vi "Transaction.vi"(8 "Error In":errorcluster, 9 "Bytes to read (1024)":u32=1024, 10 "Command":string, 11 "VISA resource name":refnum<visa-resource-name>) -> (0 "Error Out":errorcluster, 2 "Response":string, 3 "VISA resource name out":refnum<visa-resource-name>)   [LabVIEW 2013, in "HadCon.lvlib"]
doc: "This VI performs low level command /response formatting.\nThis transaction sends a command and waits for the corresponding response of the instrument."
uses:
  <instrlib>/HadCon/HadCon.lvlib
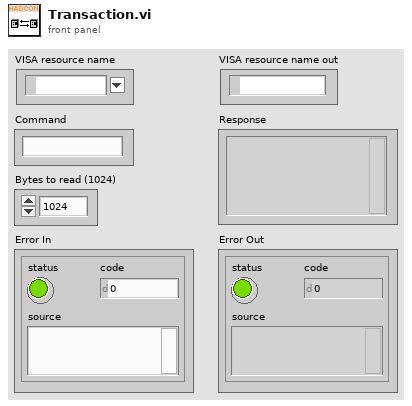
[diagram p1: front panel]
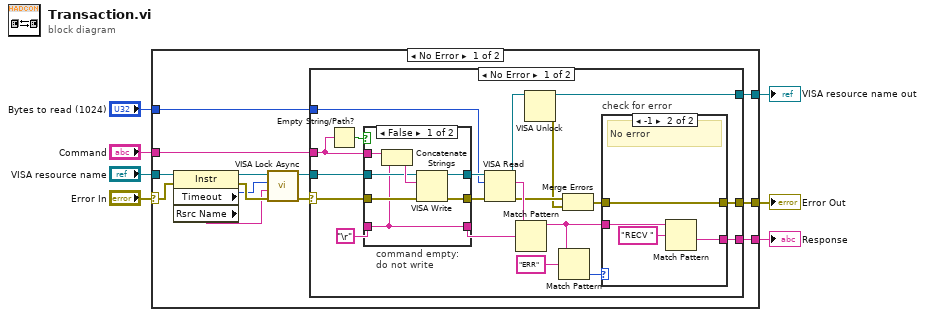
[diagram p0: block diagram]
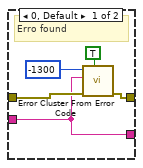
[diagram p3: hidden frame]
diagram:
  n1 = case shown="No Error" "Error In" {
    selector: "Error In" -> [w12 w63]
    tunnel: "VISA resource name" -> [w15 w62]
    tunnel: "Command" -> [w20 _]
    tunnel: "Bytes to read (1024)" -> [w19 _]
    tunnel: [w18 w62] -> w4
    tunnel: [w17 w63] -> w3
    tunnel: [w16 _] -> w2
    frame No Error {
      n2 = property class="Instr"(reference=w15, error in=w12) -> (reference out=w13:refnum<visa-resource-name>, error out=w11:errorcluster, "Timeout"=w10:u32, "Rsrc Name"=w9:string)
      n3 = call <vilib>:"VISA Lock Async.vi"("error in (no error)"=w11, "requested key"=w9, "timeout (0)"=w10, "VISA resource name"=w13) -> ("error out"=w8:errorcluster, "VISA resource name out"=w14:refnum<visa-resource-name>)  [unwired: 5 in, 1 out]
      n4 = case shown="No Error" w8 {
        selector: w8 -> [w30 w60]
        tunnel: w20 -> [w25 _]
        tunnel: w19 -> [w38 _]
        tunnel: [w28 w61] -> w18
        tunnel: [w33 w60] -> w17
        tunnel: [w32 _] -> w16
        tunnel: w14 -> [w31 w61]
        frame No Error {
          n5 = Empty String/Path?(string/path=w25) -> (empty?=w26:bool)
          n6 = case "command empty:\ndo not write" shown="False" w26 {
            tunnel: w25 -> [w41 _]
            tunnel: [w46 w50] -> w40
            tunnel: [w45 w49] -> w39
            tunnel: [w42 w48] -> w36
            tunnel: w31 -> [w44 w50]
            tunnel: w30 -> [w43 w49]
            tunnel: "\r" -> [w42 w48]
            frame False {
              n7 = Concatenate Strings(w41, w42) -> (w47:string)
              n8 = VISA Write(VISA resource name=w44, write buffer=w47, error in (no error)=w43) -> (VISA resource name out=w46:refnum<visa-resource-name>, error out=w45:errorcluster)  [unwired: 1 out]
            }
            frame True {
            }
          }
          n9 = VISA Read(VISA resource name=w40, byte count=w38, error in (no error)=w39) -> (VISA resource name out=w29:refnum<visa-resource-name>, read buffer=w37:string, error out=w23:errorcluster)  [unwired: 1 out]
          n10 = Match Pattern(string=w37, regular expression=w36) -> (before substring=w27:string)  [unwired: 1 in, 3 out]
          n11 = VISA Unlock(11:w29) -> (0:w21:errorcluster, 3:w28:refnum<visa-resource-name>)  [unwired: 1 in]
          n12 = Match Pattern(string=w27, regular expression="ERR") -> (offset past match=w34:i32)  [unwired: 1 in, 3 out]
          n13 = Merge Errors(w23, w21) -> (w22:errorcluster)
          n14 = case "check for error" shown="-1" w34 {
            tunnel: w27 -> [w51 w57]
            tunnel: w22 -> [w55 w59]
            tunnel: [w54 w59] -> w33
            tunnel: [w51 w56] -> w32
            frame 0, Default {
              # "Erro found"
              n15 = call <vilib>:"Error Cluster From Error Code.vi"("show call chain? (False)"=TRUE, "error in (no error)"=w55, "error message (\"\")"=w51, "error code (0)"=-1300) -> ("error out"=w54:errorcluster)  [unwired: 5 in]
            }
            frame -1 {
              # "No error"
              n16 = Match Pattern(string=w57, regular expression="RECV ") -> (after substring=w56:string)  [unwired: 1 in, 3 out]
            }
          }
        }
        frame Error {
        }
      }
    }
    frame Error {
    }
  }
  "Error Out" <- w3
  "VISA resource name out" <- w4
  "Response" <- w2
